vi "Wait For Operation Complete.vi"(8 "error in (no error)":errorcluster, 10 "Maximum Time (10000 ms)":i32=10000, 11 "VISA resource name":refnum<visa-resource-name>) -> (0 "error out":errorcluster, 3 "VISA resource name out":refnum<visa-resource-name>)   [LabVIEW 2019, in "Agilent 681x Series.lvlib"]
doc: "This low-level VI waits for the current measurement to complete before letting execution to continue. This VI should be called after <B>Initiate</B> VI.\n\n<B>Note:</B>\n\nUse this VI only with other low-level VIs. The high-level VIs automatically incorporate this functionality. This VI does not check the instrument status. If you want to check the instrument status, call the Error Query VI at the conclusion of the sequence.\n\nWaiting will start immediately after the VI is called regardless of receiving or not receiving a trigger."
uses:
  <instrlib>/Agilent 681x Series/Agilent 681x Series.lvlib
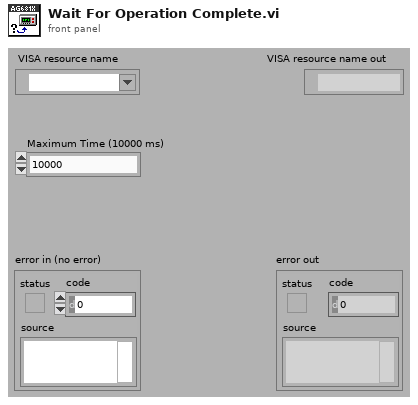
[diagram p1: front panel]
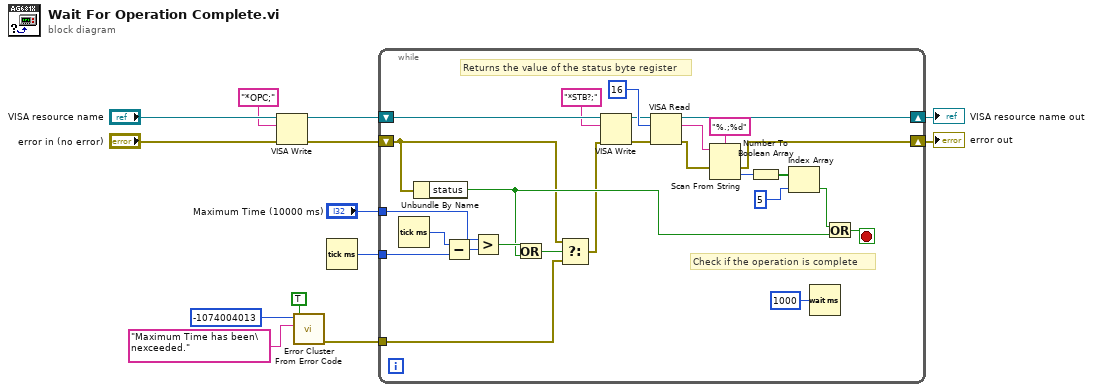
[diagram p0: block diagram]
diagram:
  n1 = VISA Write(VISA resource name="VISA resource name", write buffer="*OPC;", error in (no error)="error in (no error)") -> (VISA resource name out=w2:refnum<visa-resource-name>, error out=w1:errorcluster)  [unwired: 1 out]
  n2 = call <vilib>:"Error Cluster From Error Code.vi"("show call chain? (False)"=TRUE, "error message (\"\")"="Maximum Time has been\nexceeded." ("error message (\"\")"), "error code (0)"=-1074004013) -> ("error out"=w8:errorcluster)  [unwired: 6 in]
  n3 = Tick Count (ms)() -> (millisecond timer value=w12:u32)
  n4 = while {
    tunnel: "Maximum Time (10000 ms)" -> [w26]
    tunnel: w12 -> [w34]
    tunnel: w8 -> [w21]
    shift-right: [w32] -> w6
    shift-left: w1 -> [w20]
    shift-right: [w37] -> w7
    shift-left: w2 -> [w16]
    stop <- w27 stop-if-true
    # "Check if the operation is complete"
    # "Returns the value of the status byte register"
    n5 = Tick Count (ms)() -> (millisecond timer value=w35:u32)
    n6 = Unbundle By Name(w20) -> ("status"=w22:bool)
    n7 = Subtract(x=w35, y=w34) -> (x-y=w25:u32)
    n8 = Greater?(x=w26, y=w25) -> (0:w24:bool)
    n9 = Or(x=w24, y=w22) -> (x .or. y?=w23:bool)
    n10 = Select(t=w20, s=w23, f=w21) -> (s? t:f=w15:errorcluster)
    n11 = VISA Write(VISA resource name=w16, write buffer="*STB?;", error in (no error)=w15) -> (VISA resource name out=w18:refnum<visa-resource-name>, error out=w17:errorcluster)  [unwired: 1 out]
    n12 = VISA Read(VISA resource name=w18, byte count=u32 16, error in (no error)=w17) -> (VISA resource name out=w37:refnum<visa-resource-name>, read buffer=w39:string, error out=w33:errorcluster)  [unwired: 1 out]
    n13 = Scan From String(format string="%.;%d", input string=w39, error in=w33) -> (error out=w32:errorcluster, output 1=w29:i32)  [unwired: 2 in, 2 out]
    n14 = Number To Boolean Array(number=w29) -> (Boolean array=w30:bool[])
    n15 = Index Array(array=w30, index=5) -> (element=w28:bool)
    n16 = Wait (ms)(milliseconds to wait=u32 1000) -> ()  [unwired: 1 out]
    n17 = Or(x=w28, y=w22) -> (x .or. y?=w27:bool)
  }
  "error out" <- w6
  "VISA resource name out" <- w7
